vi "Check Subnet Strings.vi"(8 "error in (no error)":errorcluster, 9 "Mask":string, 10 "Address 2":string, 11 "Address 1":string) -> (0 "error out":errorcluster, 3 "In Subnet":bool)   [LabVIEW 2021, in "Networking_CIF_U.lvlib"]
uses:
  Networking_CIF_U.lvlib
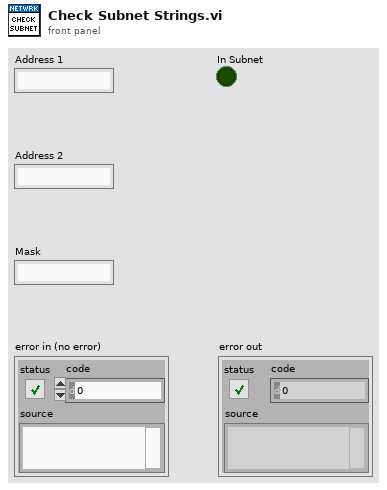
[diagram p1: front panel]
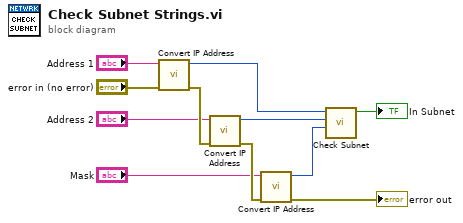
[diagram p0: block diagram]
diagram:
  n1 = call "Convert IP Address.vi"("error in (no error)"="error in (no error)", "IP"="Address 1") -> ("error out"=w8:errorcluster, "net address"=w9:u32)  [unwired: 8 in]
  n2 = call "Convert IP Address.vi"("error in (no error)"=w8, "IP"="Address 2") -> ("error out"=w7:errorcluster, "net address"=w2:u32)  [unwired: 8 in]
  n3 = call "Convert IP Address.vi"("error in (no error)"=w7, "IP"="Mask") -> ("error out"=→"error out":errorcluster, "net address"=w1:u32)  [unwired: 8 in]
  n4 = call "Check Subnet.vi"("Mask"=w1, "Address 2"=w2, "Address 1"=w9) -> ("In Subnet"=→"In Subnet":bool)  [unwired: 8 in]
